vi "onCreateListener.vi"(6 "timeout (ms)":i32=100, 8 "error in (no error)":errorcluster, 10 "Configuration":refnum<class "Connection.TCP.lvclass">) -> (0 "error out":errorcluster, 3 "Listener":refnum<class "Connection.lvclass">)   [LabVIEW 2013, in "Connection.TCP_GOSPL.lvlib" / "Connection.TCP.lvclass"]
uses:
  Connection.TCP.lvclass
  Connection/Connection.lvclass
  Connection.TCP.lvclass/Connection.TCP.ctl
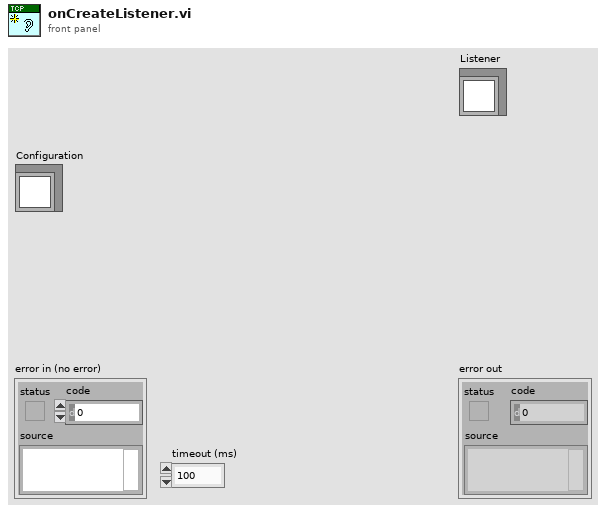
[diagram p1: front panel]
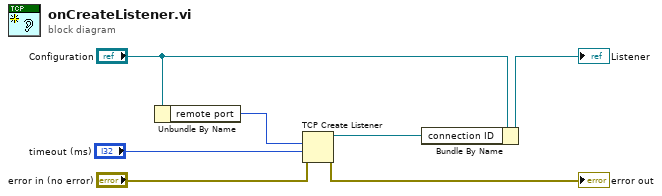
[diagram p0: block diagram]
diagram:
  n1 = Unbundle By Name("Configuration") -> ("remote port"=w4:u16)
  n2 = TCP Create Listener(8:"error in (no error)", 9:"timeout (ms)", 10:w4) -> (0:→"error out":errorcluster, 3:w6:refnum<k5>)  [unwired: 2 in, 1 out]
  n3 = Bundle By Name(cluster="Configuration", "connection ID"=w6) -> (→"Listener":refnum<class "Connection.TCP.lvclass">)
